vi "Write data.vi"(8 "error in (no error)":errorcluster, 10 "data":string, 11 "SimpleStringMessage in":refnum<class "SimpleStringMessage.lvclass">) -> (0 "error out":errorcluster, 3 "SimpleStringMessage out":refnum<class "SimpleStringMessage.lvclass">)   [LabVIEW 2013, in "SimpleStringMessage.lvclass"]
doc: "Set string data of the message"
uses:
  SimpleStringMessage.lvclass
  SimpleStringMessage.lvclass/SimpleStringMessage.ctl
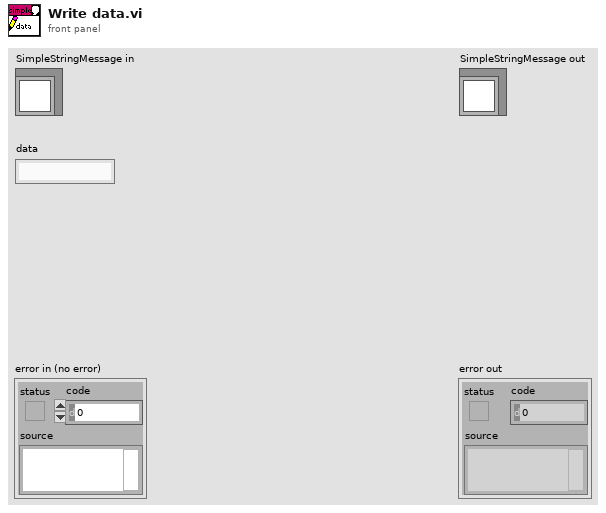
[diagram p1: front panel]
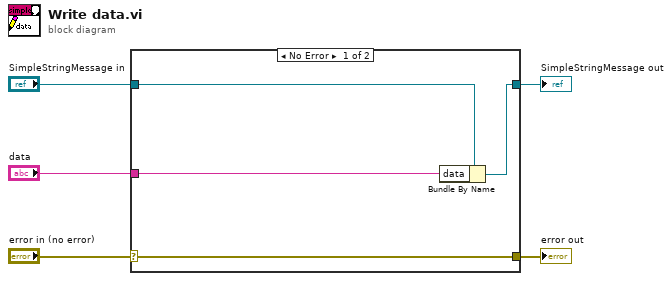
[diagram p0: block diagram]
diagram:
  n1 = case shown="No Error" "error in (no error)" {
    selector: "error in (no error)" -> [w9 w10]
    tunnel: [w9 w10] -> w4
    tunnel: [w7 w11] -> w2
    tunnel: "SimpleStringMessage in" -> [w8 w11]
    tunnel: "data" -> [w6 _]
    frame No Error {
      n2 = Bundle By Name(cluster=w8, "data"=w6) -> (w7:refnum<class "SimpleStringMessage.lvclass">)
    }
    frame Error {
    }
  }
  "error out" <- w4
  "SimpleStringMessage out" <- w2
